vi "Status Read Start.vi"(8 "error in (no error)":errorcluster, 11 "Status Reference":T1) -> (0 "error out":errorcluster, 1 "Start":bool, 3 "Status Reference out":T1)   [LabVIEW 2021, in "Status.lvlib"]
uses:
  Status.lvlib
  Ctl/control.ctl
  Ctl/State.ctl
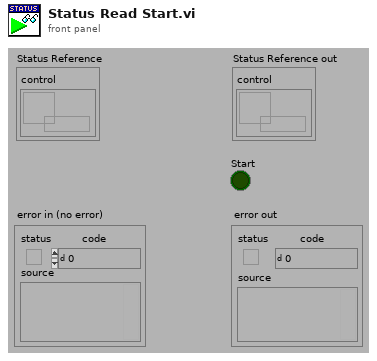
[diagram p1: front panel]
types:
  T1 = typedef "Status.lvlib/control.ctl" = cluster{"control":refnum<data-value>}
  T2 = typedef "Status.lvlib/State.ctl" = enum8{"initialization", "redefine", "standby", "connect", "wait to reconnect", "wait to reset timeout", "configure", "requests", "close connection", "stop"}
  T3 = cluster{"set_state":cluster{"Start":bool, "WrEn":bool, "Stop":bool}, "state":cluster{"errors":i32, "connect":bool, "state":T2}}
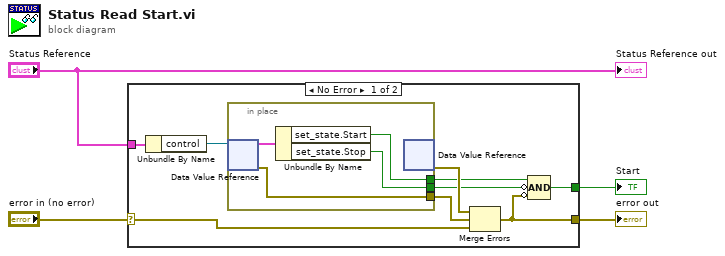
[diagram p0: block diagram]
diagram:
  n1 = case shown="No Error" "error in (no error)" {
    selector: "error in (no error)" -> [w9 w18]
    tunnel: [w7 w18] -> w4
    tunnel: [w6 _] -> w3
    tunnel: "Status Reference" -> [w13 _]
    frame No Error {
      n2 = Unbundle By Name(w13) -> ("control"=w11:refnum<data-value>)
      n3 = in-place {
        in-place-border: [w17] -> w10
        in-place-border: [w15] -> w8
        in-place-border: [w14] -> w5
        n4 = in-place-dvr #1(w11) -> (w16:T3, w17:errorcluster)
        n5 = Unbundle By Name(w16) -> ("set_state.Start"=w15:bool, "set_state.Stop"=w14:bool)
        n6 = in-place-dvr #1() -> (w12:errorcluster)  [unwired: 1 in, 1 out]
      }
      n7 = Merge Errors(w12, w10, w9) -> (w7:errorcluster)
      n8 = Compound Arithmetic op=AND(w8, invert w5, invert w7) -> (w6:bool)
    }
    frame Error {
    }
  }
  "error out" <- w4
  "Start" <- w3
  "Status Reference out" <- "Status Reference"
